vi "Restore Window.vi"(4 "error in (no error)":errorcluster, 6 "window name  (\"\")":string, 7 "window refnum (NaWR)":T1) -> (0 "error out":errorcluster, 3 "window refnum out":T1)   [LabVIEW 2023, in "WINUTIL.lvlib"]
doc: "This function will restore the window named in the window name input if the window refnum supplied is invalid, otherwise it uses window refnum to determine which window is restored. If the window cannot be found, an error will be returned."
uses:
  WINUTIL.lvlib
  Window Refnum.ctl
  LVWUtil32.dll
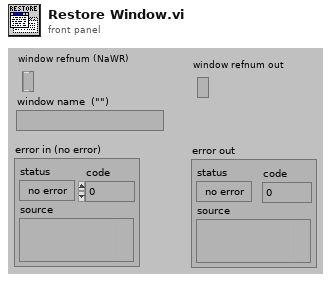
[diagram p1: front panel]
types:
  T1 = typedef "WINUTIL.lvlib/Window Refnum.ctl" = refnum<k1>
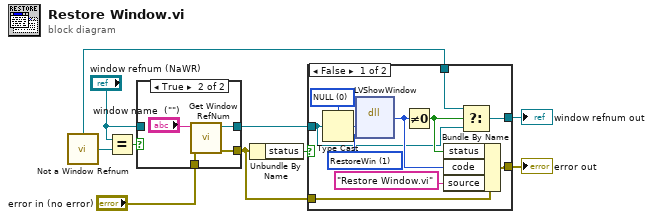
[diagram p0: block diagram]
diagram:
  n1 = call "Not a Window Refnum.vi"() -> ("Not a Window Refnum"=w4:T1)
  n2 = Equal?(x="window refnum (NaWR)", y=w4) -> (x = y?=w2:bool)
  n3 = case shown="True" w2 {
    tunnel: "error in (no error)" -> [w10 w15]
    tunnel: [w11 w14] -> w5
    tunnel: "window refnum (NaWR)" -> [w11 _]
    tunnel: [w10 w13] -> w7
    frame False {
    }
    frame True {
      n4 = call "Get Window RefNum.vi"("error in (no error)"=w15, "window name (\"\")"="window name  (\"\")") -> ("error out"=w13:errorcluster, "window refnum (NaWR)"=w14:T1)  [unwired: 6 out]
    }
  }
  n5 = Unbundle By Name(w7) -> ("status"=w8:bool)
  n6 = case shown="False" w8 {
    tunnel: w7 -> [w21 w28]
    tunnel: [w25 w28] -> w6
    tunnel: w5 -> [w17 w27]
    tunnel: [w16 w27] -> w1
    tunnel: w4 -> [w20 _]
    frame False {
      w26 = u8 1 items=["ShowWindow", "RestoreWin"]
      w18 = u32 0 items=["NULL"]
      n7 = Type Cast(type=w18, x=w17) -> (*(type *) &x=w19:u32)
      n8 = dll-call lib="C:/Users/acasalen/Documents/LabVIEW Data/Projects/Reds-Auto-Clicker/Red's Auto Clicker/SubVIs/labview_win_util32_8.6/lvwutil32.dll" fn="LVShowWindow"("hWnd"=w19, "function"=w26) -> ("error"=w24:i32)  [unwired: 5 in, 2 out]
      n9 = Not Equal To 0?(x=w24) -> (x != 0?=w23:bool)
      n10 = Bundle By Name(cluster=w21, "status"=w23, "code"=w24, "source"="Restore Window.vi") -> (w25:errorcluster)
      n11 = Select(t=w20, s=w23, f=w17) -> (s? t:f=w16:T1)
    }
    frame True {
    }
  }
  "error out" <- w6
  "window refnum out" <- w1
